vi "MoveLineNumbers.vi"(8 "Force?":bool, 11 "Refs":T1) -> ()   [LabVIEW 2020, in "Code.xctl"]
uses:
  <vilib>/Utility/miscctls.llb/LVSelectionTypeDef.ctl
  ColorGlobals.vi
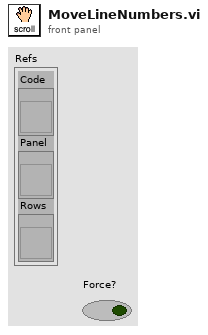
[diagram p1: front panel]
types:
  T1 = cluster{"Code":refnum<vi>, "Panel":refnum<vi>, "Rows":refnum<vi>}
  T2 = typedef "LVSelectionTypeDef.ctl" = cluster{"Selection Start":u32, "Selection End":u32}
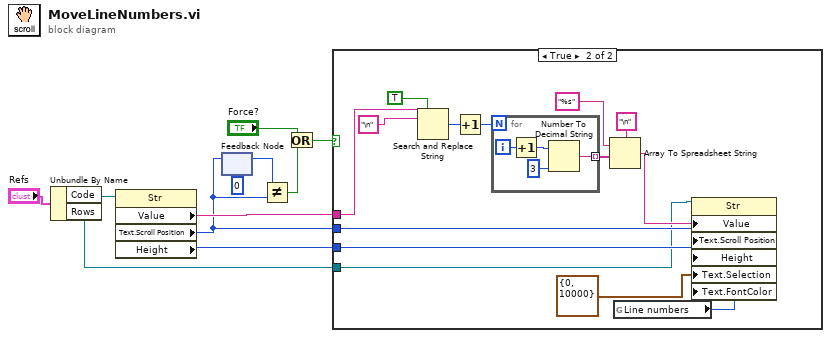
[diagram p0: block diagram]
diagram:
  n1 = Unbundle By Name("Refs") -> ("Code"=w2:refnum<vi>, "Rows"=w1:refnum<vi>)
  n2 = property on="Property Node" class="Str"(reference=w2) -> ("Value"=w9:string, "Text.Scroll Position"=w7:u32, "Height"=w10:u32)  [unwired: 1 in, 2 out]
  n3 = feedback-in #1(w7) -> ()
  n4 = feedback #1(u32 0 ("Text.Scroll Position")) -> (w8:u32)
  n5 = Not Equal?(x=w8, y=w7) -> (x != y?=w4:bool)
  n6 = Or(x="Force?", y=w4) -> (x .or. y?=w3:bool)
  n7 = case shown="True" w3 {
    tunnel: w10 -> [_ w21]
    tunnel: w9 -> [_ w17]
    tunnel: w7 -> [_ w15]
    tunnel: w1 -> [_ w14]
    frame False {
    }
    frame True {
      n8 = Search and Replace String(replace all?=TRUE ("replace all? (F)"), input string=w17, search string="\n") -> (number of replacements=w18:i32)  [unwired: 5 in, 3 out]
      n9 = Increment(x=w18) -> (x+1=w20:i32)
      n10 = for {
        N: w20 -> [_]
        tunnel: [w29] -> w19 mode=indexing
        i -> [w26]
        n11 = Increment(x=w26) -> (x+1=w28:i32)
        n12 = Number To Decimal String(number=w28, width (-)=i16 3) -> (decimal integer string=w29:string)
      }
      n13 = Array To Spreadsheet String(delimiter (Tab)="\n", array=w19, 3:"%s" ("format string")) -> (spreadsheet string=w16:string)
      n14 = global read "ColorGlobals.vi" "Line numbers"() -> (w12:u32)
      n15 = property on="Property Node" class="Str"(reference=w14, "Value"=w16, "Text.Scroll Position"=w15, "Height"=w21, "Text.Selection"=T2 {"Selection Start"=0, "Selection End"=10000}, "Text.FontColor"=w12) -> ()  [unwired: 1 in, 2 out]
    }
  }
